vi "Initialize.vi"(8 "error in (no error)":errorcluster, 9 "Reset (True)":bool, 10 "ID Query (True)":bool=TRUE, 11 "VISA resource name":refnum<visa-resource-name>) -> (0 "error out":errorcluster, 3 "VISA resource name out":refnum<visa-resource-name>)   [LabVIEW 2024, in "EFmeter.lvlib"]
doc: "Establishes communication with the instrument and optionally performs an instrument identification query and/or an instrument reset. It also places the instrument in a default state needed for other instrument driver operations. Therefore, call this VI before calling other instrument driver VIs for this instrument. Generally, you need to call the <b>Initialize</b> VI only once at the beginning of an application."
uses:
  <instrlib>/EFmeter/EFmeter.lvlib
panel:
  in  "Serial Configuration":T1={"Baud Rate"=115200, "Parity"=0, "Data Bits"=8, "Stop Bits"=10, "Flow Control"=0} {"Flow Control" items=["None", "XON/XOFF", "RTS/CTS", "XON/XOFF & RTS/CTS", "DTR/DSR", "XON/XOFF & DTR/DSR"]; "Stop Bits" items=["1.0"=10, "1.5"=15, "2.0"=20]; "Data Bits" items=["7"=7, "8"=8]; "Parity" items=["None", "Odd", "Even", "Mark", "Space"]; "Baud Rate" items=["300"=300, "600"=600, "1200"=1200, "2400"=2400, "4800"=4800, "9600"=9600, "19200"=19200]}
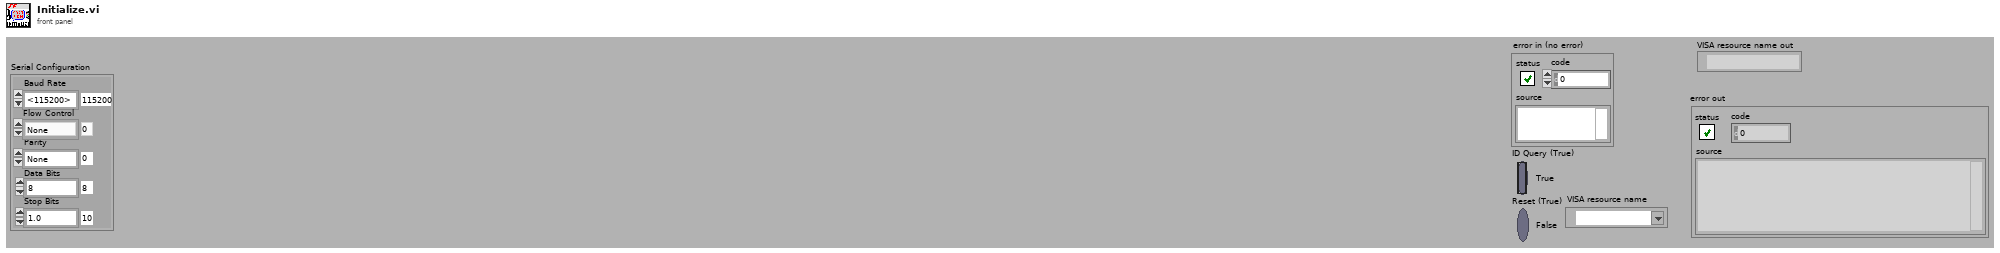
[diagram p1: front panel]
types:
  T1 = cluster{"Baud Rate":u32, "Parity":u16, "Data Bits":u16, "Stop Bits":u16, "Flow Control":u16}
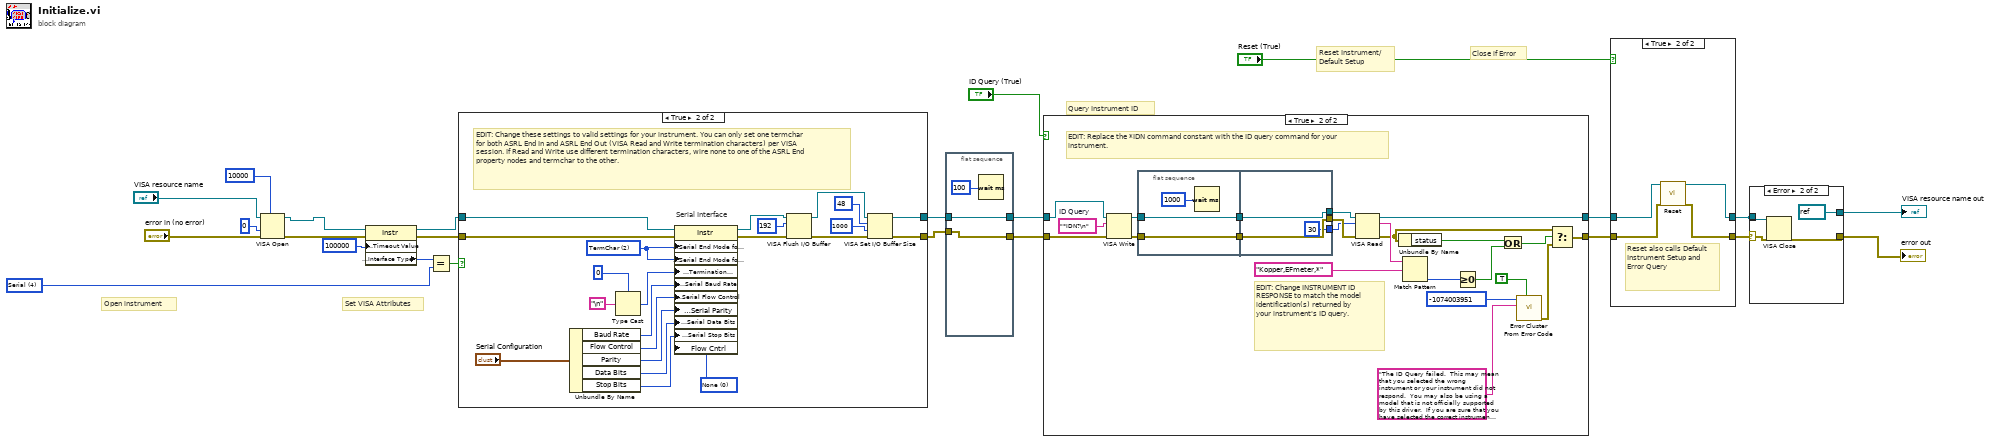
[diagram p0: block diagram]
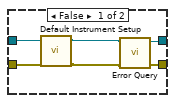
[diagram p4: hidden frame]
diagram:
  w13 = u16 4 items=["GPIB"=1, "VXI"=2, "GPIB-VXI"=3, "Serial"=4, "PXI"=5, "TCPIP"=6, "USB"=7] ("Interface Information:Interface Type")
  # "Set VISA Attributes"
  # "Close if Error"
  # "Query Instrument ID"
  # "Reset Instrument/\nDefault Setup"
  # "Open instrument"
  n1 = VISA Open(timeout (0)=u32 10000 ("VISA Open timeout (0)"), access mode=u32 0, error in (no error)="error in (no error)", VISA resource name="VISA resource name") -> (VISA resource name=w3:refnum<visa-resource-name>, error out=w2:errorcluster)  [unwired: 1 in]
  n2 = property class="Instr"(reference=w3, error in=w2, "General Settings:Timeout Value"=u32 100000) -> (reference out=w16:refnum<visa-resource-name>, error out=w15:errorcluster, "Interface Information:Interface Type"=w18:u16)
  n3 = Equal?(x=w18, y=w13) -> (x = y?=w14:bool)
  n4 = case shown="True" w14 {
    tunnel: [w25 w45] -> w9
    tunnel: [w26 w42] -> w6
    tunnel: w16 -> [w25 w47]
    tunnel: w15 -> [w26 w48]
    frame False {
      # "EDIT: Remove interfaces not supported by your instrument."
      # "GPIB, TCP/IP, and USB Interface"
    }
    frame True {
      w27 = u16 0 items=["None", "XON/XOFF", "RTS/CTS", "XON/XOFF & RTS/CTS", "DTR/DSR", "XON/XOFF & DTR/DSR"] ("Serial Settings:Flow Control")
      w35 = u16 2 items=["None", "LastBit", "TermChar"] ("Serial Settings:Serial End Mode for Reads")
      # "EDIT: Change these settings to valid settings for your instrument. You can only set one termchar for both ASRL End In and ASRL End Out (VISA Read and Write termination characters) per VISA session. If Read and Write use different termination characters, wire none to one of the ASRL End property nodes and termchar to the other."
      # "Serial Interface"
      n5 = Unbundle By Name("Serial Configuration") -> ("Baud Rate"=w33:u32, "Flow Control"=w29:u16, "Parity"=w31:u16, "Data Bits"=w32:u16, "Stop Bits"=w28:u16)
      n6 = Type Cast(type=u8 0, x="\n" ("Line Feed Constant")) -> (*(type *) &x=w34:u8)
      n7 = property class="Instr"(reference=w47, error in=w48, "Serial Settings:Serial End Mode for Reads"=w35, "Serial Settings:Serial End Mode for Writes"=w35, "Message Based Settings:Termination Character"=w34, "Serial Settings:Serial Baud Rate"=w33, "Serial Settings:Serial Flow Control"=w29, "Serial Settings:Serial Parity"=w31, "Serial Settings:Serial Data Bits"=w32, "Serial Settings:Serial Stop Bits"=w28, "Flow Cntrl"=w27) -> (reference out=w41:refnum<visa-resource-name>, error out=w44:errorcluster)
      n8 = VISA Flush I/O Buffer(VISA resource name=w41, mask (16)=u16 192, error in (no error)=w44) -> (VISA resource name out=w46:refnum<visa-resource-name>, error out=w43:errorcluster)
      n9 = VISA Set I/O Buffer Size(VISA resource name=w46, mask (16)=u16 48, size (4096)=u32 1000 ("size (0)"), error in (no error)=w43) -> (VISA resource name out=w45:refnum<visa-resource-name>, error out=w42:errorcluster)
    }
  }
  n10 = flat-sequence {
    tunnel: w9 -> [w51]
    tunnel: [w51] -> w8
    tunnel: [w50] -> w7
    tunnel: w6 -> [w50]
    frame #0 {
      n11 = Wait (ms)(milliseconds to wait=u32 100) -> ()  [unwired: 1 out]
    }
  }
  n12 = case shown="True" "ID Query (True)" {
    tunnel: [w52 w76] -> w23
    tunnel: [w53 w73] -> w24
    tunnel: w8 -> [w53 w74]
    tunnel: w7 -> [w52 w75]
    frame False {
    }
    frame True {
      w70 = "*IDN?\n"  # ID Query
      # "EDIT: Replace the *IDN command constant with the ID query command for your instrument."
      # "EDIT: Change INSTRUMENT ID RESPONSE to match the model identification(s) returned by your instrument's ID query."
      n13 = VISA Write(VISA resource name=w74, write buffer=w70, error in (no error)=w75) -> (VISA resource name out=w59:refnum<visa-resource-name>, error out=w60:errorcluster)  [unwired: 1 out]
      n14 = flat-sequence {
        tunnel: w60 -> [w79]
        tunnel: w59 -> [w78]
        tunnel: [w79] -> w58
        tunnel: [w78] -> w57
        tunnel: w58 -> [w81]
        tunnel: w57 -> [w82]
        tunnel: [w82] -> w56
        tunnel: [w81] -> w55
        tunnel: [u32 30 ("Bytes at Port")] -> w54
        frame #0 {
          n15 = Wait (ms)(milliseconds to wait=u32 1000) -> ()  [unwired: 1 out]
        }
        frame #1 {
        }
      }
      n16 = VISA Read(VISA resource name=w56, byte count=w54, error in (no error)=w55) -> (VISA resource name out=w73:refnum<visa-resource-name>, read buffer=w72:string, error out=w64:errorcluster)  [unwired: 1 out]
      n17 = Unbundle By Name(w64) -> ("status"=w63:bool)
      n18 = Match Pattern(string=w72, regular expression="Kopper,EFmeter,*") -> (offset past match=w65:i32)  [unwired: 1 in, 3 out]
      n19 = Greater Or Equal To 0?(x=w65) -> (x >= 0?=w62:bool)
      n20 = Or(x=w63, y=w62) -> (x .or. y?=w61:bool)
      n21 = call <vilib>:"Error Cluster From Error Code.vi"("show call chain? (False)"=TRUE, "error message (\"\")"="The ID Query failed.  This may mean that you selected the wrong instrument or your instrument did not respond.  You may also be using a model that is not officially supported by this driver.  If you are sure that you have selected the correct instrument and it is responding, try disabling the ID Query." ("Source (VI Name)"), "error code (0)"=-1074003951 ("Code")) -> ("error out"=w69:errorcluster)  [unwired: 6 in]
      n22 = Select(t=w64, s=w61, f=w69) -> (s? t:f=w76:errorcluster)
    }
  }
  n23 = case shown="True" "Reset (True)" {
    tunnel: w23 -> [w83 w91]
    tunnel: [w88 w90] -> w4
    tunnel: w24 -> [w84 w92]
    tunnel: [w87 w89] -> w1
    frame False {
      n24 = call <instrlib>:"Default Instrument Setup.vi"("error in (no error)"=w83, "VISA resource name"=w84) -> ("error out"=w85:errorcluster, "VISA resource name out"=w86:refnum<visa-resource-name>)  [unwired: 8 in]
      n25 = call <instrlib>:"Error Query.vi"("error in (no error)"=w85, "VISA resource name"=w86) -> ("error out"=w88:errorcluster, "VISA resource name out"=w87:refnum<visa-resource-name>)  [unwired: 6 in, 2 out]
    }
    frame True {
      # "Reset also calls Default Instrument Setup and Error Query"
      n26 = call <instrlib>:"Reset.vi"("error in (no error)"=w91, "VISA resource name"=w92) -> ("error out"=w90:errorcluster, "VISA resource name out"=w89:refnum<visa-resource-name>)  [unwired: 8 in]
    }
  }
  n27 = case shown="Error" w4 {
    selector: w4 -> [w93 w97]
    tunnel: w1 -> [w94 w96]
    tunnel: [w94 refnum<visa-resource-name> refnum ("VISA resource name out")] -> w11
    tunnel: [w93 w95] -> w10
    tunnel: w1 -> [_ _]
    frame No Error {
    }
    frame Error {
      n28 = VISA Close(VISA resource name=w96, error in (no error)=w97) -> (error out=w95:errorcluster)
    }
  }
  "VISA resource name out" <- w11
  "error out" <- w10
